vi "Time.DateTime Limit.vi"(7 "LimitHrs":dbl=24.0, 10 "End":timestamp, 11 "Start":timestamp) -> (2 "End Out":timestamp, 3 "Start Out":timestamp)   [LabVIEW 2019]
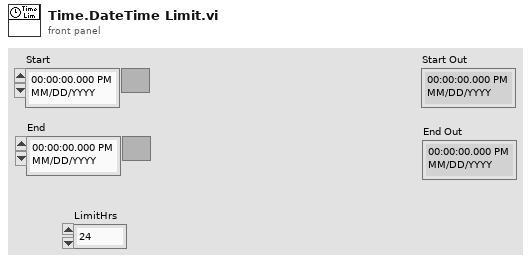
[diagram p1: front panel]
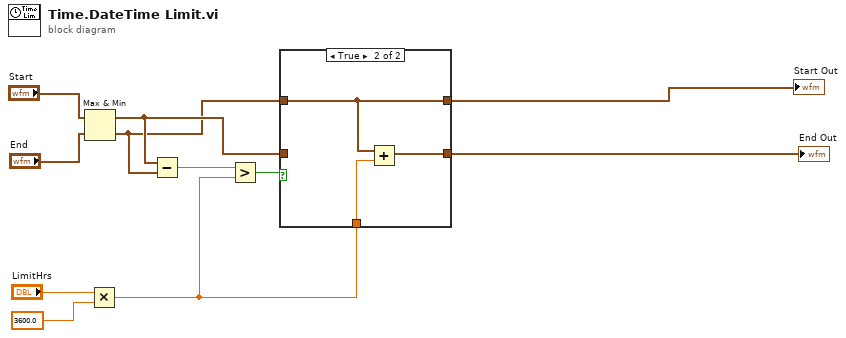
[diagram p0: block diagram]
diagram:
  n1 = Max & Min(x="Start", y="End") -> (max(x,y)=w5:timestamp, min(x,y)=w4:timestamp)
  n2 = Multiply(x="LimitHrs", y=3600.0) -> (x*y=w1:dbl)
  n3 = Subtract(x=w5, y=w4) -> (x-y=w7:dbl)
  n4 = Greater?(x=w7, y=w1) -> (0:w6:bool)
  n5 = case shown="True" w6 {
    tunnel: w5 -> [w12 _]
    tunnel: w4 -> [w13 w14]
    tunnel: [w13 w14] -> w3
    tunnel: [w12 w15] -> w2
    tunnel: w1 -> [_ w16]
    frame False {
    }
    frame True {
      n6 = Add(x=w14, y=w16) -> (x+y=w15:timestamp)
    }
  }
  "Start Out" <- w3
  "End Out" <- w2
